vi "Create UDP Error.vi"(9 "source vi name":string, 11 "Error":T1) -> (1 "offset":i32, 3 "error out":errorcluster)   [LabVIEW 2017, in "UDP.lvlib" / "UDP Transceiver.lvclass"]
uses:
  UDP Transceiver.lvclass
  Errors.ctl
  Library Name.vi
  <vilib>/NI/Memory Manager/VIs/New Error Cluster (512B).vi
  <vilib>/NI/Memory Manager/Static Errors.lvlib
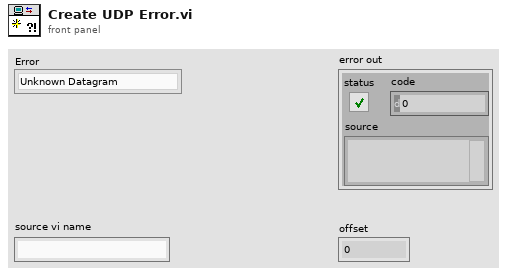
[diagram p1: front panel]
types:
  T1 = typedef "UDP.lvlib/UDP Transceiver.lvclass/Errors.ctl" = enum16{"Unknown Datagram", "Size Mismatch", "Invalid Setting"}
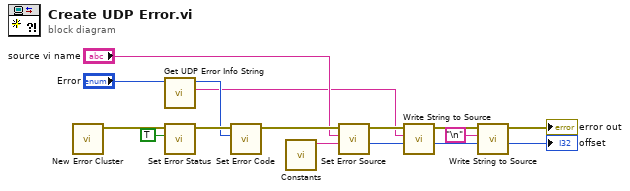
[diagram p0: block diagram]
diagram:
  n1 = call-poly <vilib>:"New Error Cluster.vi"() -> ("error out"=w15:errorcluster)  [unwired: 10 in, 1 out]
  n2 = call "Get UDP Error Info String.vi"("Error"="Error") -> ("description"=w6:string, "code"=w9:i32)  [unwired: 9 in]
  n3 = call <vilib>:"Set Error Status.vi"("status (T)"=TRUE, "error in"=w15) -> ("error out"=w13:errorcluster)  [unwired: 8 in, 1 out]
  n4 = call <vilib>:"Set Error Code.vi"("code"=w9, "error in"=w13) -> ("error out"=w12:errorcluster)  [unwired: 8 in, 1 out]
  n5 = call-poly "Constants.vi"() -> ("library name"=w10:string)  [unwired: 11 in]
  n6 = call <vilib>:"Set Error Source.vi"("library name (\"\")"=w10, "vi name"="source vi name", "error in"=w12) -> ("initial offset"=w7:i32, "error out"=w8:errorcluster)  [unwired: 7 in]
  n7 = call <vilib>:"Write String to Source.vi"("offset"=w7, "string"=w6, "error in"=w8) -> ("new offset"=w4:i32, "error out"=w5:errorcluster)  [unwired: 7 in]
  n8 = call <vilib>:"Write String to Source.vi"("offset"=w4, "string"="\n", "error in"=w5) -> ("new offset"=→"offset":i32, "error out"=→"error out":errorcluster)  [unwired: 7 in]
